vi "LVClass_CorrectionDataManager ctor from copy.vi"(0 "CorrectionDataManager in":refnum<class "CorrectionDataManager.lvclass">, 5 "CorrectionDataManager to Copy":refnum<class "CorrectionDataManager.lvclass">, 11 "error in (no error)":errorcluster) -> (4 "CorrectionDataManager out":refnum<class "CorrectionDataManager.lvclass">, 15 "error out":errorcluster)   [LabVIEW 2020, in "CorrectionDataManager.lvclass"]
doc: "CorrDataManager copy constructor.\n\n--------------------------------------------------------------------------------\n\n<B>corrdata_managerIn </B> : Constant Pointer to CorrDataManager object.\n<B>corrdata_managerOut </B> : Constant Pointer to CorrDataManager object.\n<B>corrdata_manager_src </B> : Adress of the CorrDataManager object to be copied.\n<B>ErrorIn </B> : Error\n<B>ErrorOut </B> : Error\n\n--------------------------------------------------------------------------------"
uses:
  CorrectionDataManager.lvclass
  Handle creation.ctl
  CorrectionDataManager.lvclass/CorrectionDataManager.ctl
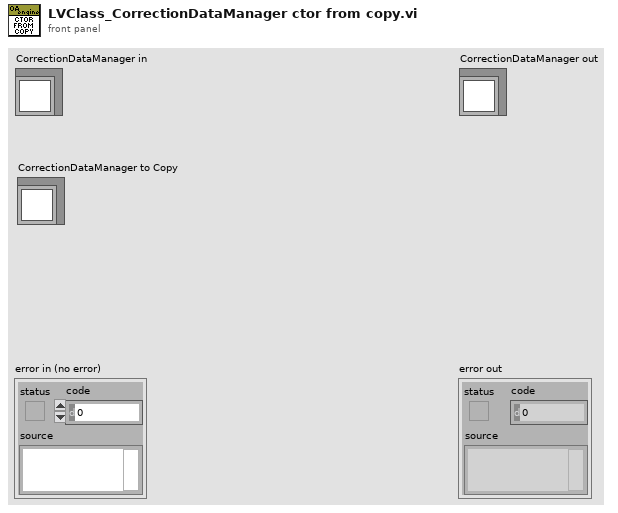
[diagram p1: front panel]
types:
  T1 = typedef "Handle creation.ctl" = enum16{"By ctor", "By write function"}
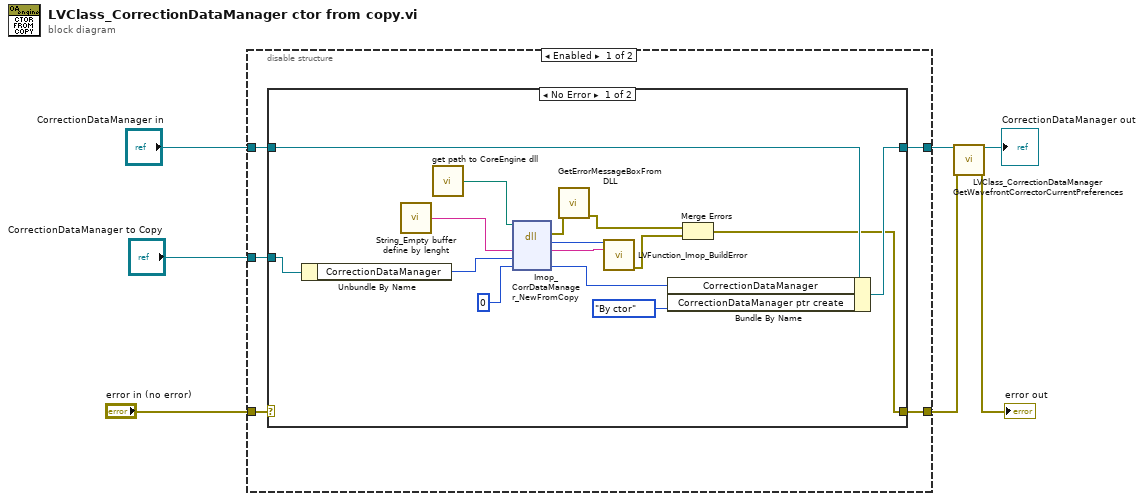
[diagram p0: block diagram]
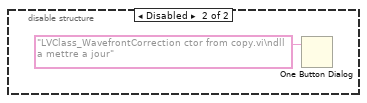
[diagram p3: hidden frame]
diagram:
  n1 = disable-structure shown="Enabled" {
    disable-tunnel: "error in (no error)" -> [w12 _]
    disable-tunnel: [w11 _] -> w3
    disable-tunnel: "CorrectionDataManager in" -> [w10 _]
    disable-tunnel: [w9 _] -> w4
    disable-tunnel: "CorrectionDataManager to Copy" -> [w8 _]
    frame Enabled {
      n2 = case shown="No Error" w12 {
        selector: w12 -> [_ w29]
        tunnel: [w13 w29] -> w11
        tunnel: [w15 w28] -> w9
        tunnel: w10 -> [w16 w28]
        tunnel: w8 -> [w17 _]
        frame No Error {
          n3 = Unbundle By Name(w17) -> ("CorrectionDataManager"=w14:i32)
          n4 = call "String_Empty buffer define by lenght.vi"() -> ("Empty buffer"=w25:string)  [unwired: 1 in]
          n5 = call "get path to CoreEngine dll.vi"() -> ("path to c_interface_vc100.dll"=w24:path)  [unwired: 12 in, 3 out]
          n6 = dll-call lib="D:/soft/HASO_v3/SVN_trunk/ImOpCoreEngine4_LV2011/DLLs/c_interface_vc100.dll" fn="Imop_CorrDataManager_NewFromCopy"(path in=w24, "message"=w25, "WavefrontCorrectionToCopy"=w14, "WavefrontCorrection"=0 ("objet")) -> (error out=w23:errorcluster, "return type"=w27:i32, "message"=w26:string, "WavefrontCorrection"=w21:i32)  [unwired: 3 in, 1 out]
          n7 = call "GetErrorMessageBoxFromDLL.vi"("error IN"=w23) -> ("error OUT"=w19:errorcluster)  [unwired: 10 in]
          n8 = call "LVFunction_Imop_BuildError.vi"("code"=w27, "String to Prepend to source (\"\")"=w26) -> ("error out"=w18:errorcluster)  [unwired: 13 in]
          n9 = Bundle By Name(cluster=w16, "CorrectionDataManager"=w21, "CorrectionDataManager ptr create"=Handle_creation."By ctor" ("HasoData ptr create")) -> (w15:refnum<class "CorrectionDataManager.lvclass">)
          n10 = Merge Errors(w19, w18) -> (w13:errorcluster)
        }
        frame Error {
        }
      }
    }
    frame Disabled {
      n11 = One Button Dialog(message="LVClass_WavefrontCorrection ctor from copy.vi\ndll a mettre a jour") -> ()  [unwired: 1 in, 1 out]
    }
  }
  n12 = call "LVClass_CorrectionDataManager GetWavefrontCorrectorCurrentPreferences.vi"("CorrectionDataManager in"=w4, "error in (no error)"=w3) -> ("CorrectionDataManager out"=→"CorrectionDataManager out":refnum<class "CorrectionDataManager.lvclass">, "error out"=→"error out":errorcluster)  [unwired: 11 in, 1 out]
